vi "Delete Folder or File if Exist.vi"(8 "error in (no error)":errorcluster, 11 "Path":path) -> (0 "error out":errorcluster, 3 "Path out":path)   [LabVIEW 2016, in "SLL File IO.lvlib"]
doc: "Deletes the file or folder if exists."
uses:
  SLL File IO.lvlib
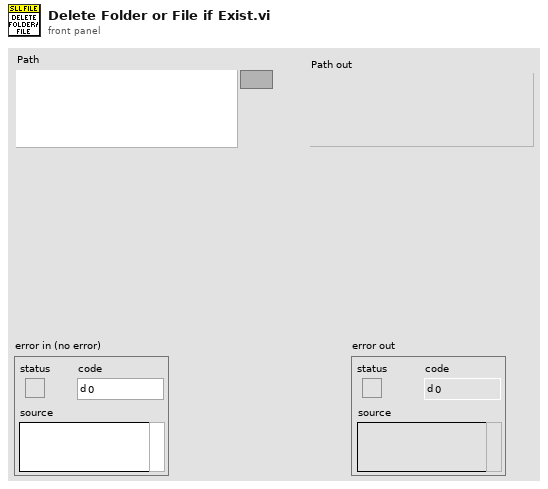
[diagram p1: front panel]
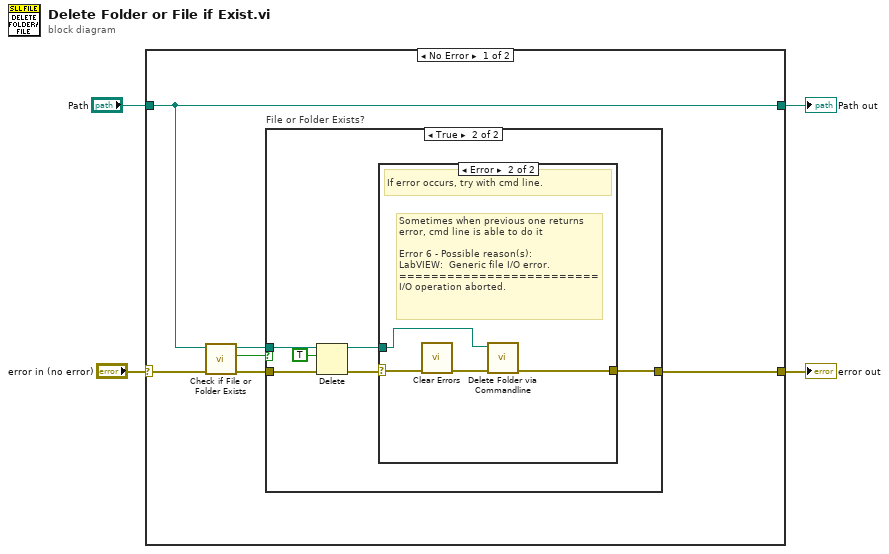
[diagram p0: block diagram]
diagram:
  n1 = case shown="No Error" "error in (no error)" {
    selector: "error in (no error)" -> [w10 w24]
    tunnel: [w9 w24] -> w3
    tunnel: "Path" -> [w5 w23]
    tunnel: [w5 w23] -> w1
    frame No Error {
      n2 = call <vilib>:"Check if File or Folder Exists.vi"("error in (no error)"=w10, "path"=w5) -> ("error out"=w8:errorcluster, "file or folder exists?"=w7:bool, "dup path"=w6:path)  [unwired: 7 in]
      n3 = case "File or Folder Exists?" shown="True" w7 {
        tunnel: [w11 w14] -> w9
        tunnel: w8 -> [w11 w17]
        tunnel: w6 -> [_ w16]
        frame False {
        }
        frame True {
          n4 = Delete(path (use dialog)=w16, entire hierarchy (F)=TRUE, error in=w17) -> (deleted path=w13:path, error out=w12:errorcluster)  [unwired: 2 in, 1 out]
          n5 = case shown="Error" w12 {
            selector: w12 -> [w18 w22]
            tunnel: [w18 w20] -> w14
            tunnel: w13 -> [_ w19]
            frame No Error {
            }
            frame Error {
              # "Sometimes when previous one returns\nerror, cmd line is able to do it\n\nError 6 - Possible reason(s):\nLabVIEW:  Generic file I/O error.\n=========================\nI/O operation aborted."
              # "If error occurs, try with cmd line."
              n6 = call <vilib>:"Clear Errors.vi"("error in (no error)"=w22) -> ("error out"=w21:errorcluster)  [unwired: 5 in, 1 out]
              n7 = call "Delete Folder via Commandline.vi"("error in (no error)"=w21, "Path"=w19) -> ("error out"=w20:errorcluster)  [unwired: 8 in, 1 out]
            }
          }
        }
      }
    }
    frame Error {
    }
  }
  "error out" <- w3
  "Path out" <- w1
